vi "SetCalcSource.vi"(8 "error in (no error)":errorcluster caption="entrée d'erreur (pas d'erreur)", 9 "DataQRefs":refnum<queue>[](array[refnum]), 10 "ScanDataQ":string[](array[string]), 11 "InstrClassIn":refnum<class "Calculations.lvclass"> caption="DNL_LabVIEW Object in") -> (0 "error out":errorcluster caption="sortie d'erreur", 3 "InstrClassOut":refnum<class "Calculations.lvclass"> caption="DNL_LabVIEW Object out")   [LabVIEW 2019, in "Calculations.lvclass"]
uses:
  Calculations.lvclass
  Calculations.lvclass/Calculations.ctl
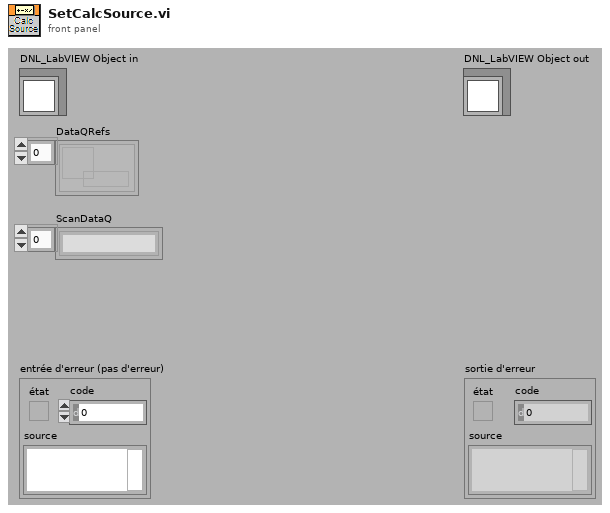
[diagram p1: front panel]
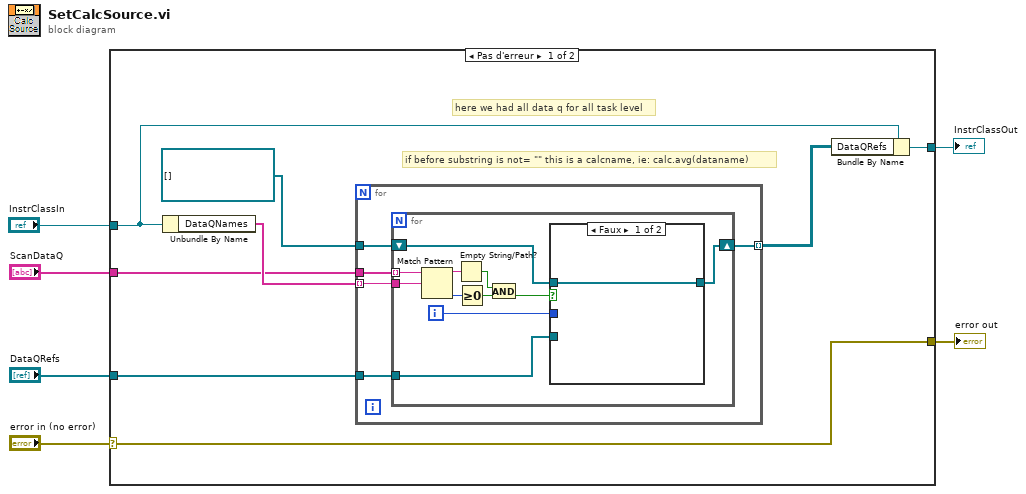
[diagram p0: block diagram]
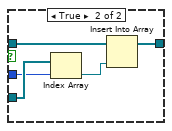
[diagram p2: hidden frame]
diagram:
  n1 = case shown="Pas d'erreur" "error in (no error)" {
    selector: "error in (no error)" -> [w7 w37]
    tunnel: "InstrClassIn" -> [w8 w38]
    tunnel: [w10 w38] -> w4
    tunnel: [w7 w37] -> w3
    tunnel: "ScanDataQ" -> [w13 _]
    tunnel: "DataQRefs" -> [w12 _]
    frame No Error {
      # "here we had all data q for all task level"
      # "if before substring is not= \"\" this is a calcname, ie: calc.avg(dataname)"
      n2 = Unbundle By Name(w8) -> ("DataQNames"=w14:string[])
      n3 = for {
        tunnel: w14 -> [w19] mode=indexing
        tunnel: w13 -> [w18]
        tunnel: w12 -> [w17]
        tunnel: refnum<queue>[] [] -> [w16]
        tunnel: [w15] -> w9 mode=indexing
        n4 = for {
          tunnel: w19 -> [w30]
          tunnel: w18 -> [w29] mode=indexing
          shift-right: [w24] -> w15
          shift-left: w16 -> [w23]
          tunnel: w17 -> [w26]
          i -> [w25]
          n5 = Match Pattern(string=w29, regular expression=w30) -> (before substring=w22:string, offset past match=w28:i32)  [unwired: 1 in, 2 out]
          n6 = Empty String/Path?(string/path=w22) -> (empty?=w20:bool)
          n7 = Greater Or Equal To 0?(x=w28) -> (x >= 0?=w27:bool)
          n8 = And(x=w20, y=w27) -> (x .and. y?=w21:bool)
          n9 = case shown="Faux" w21 {
            tunnel: w26 -> [_ w36]
            tunnel: w25 -> [_ w35]
            tunnel: [w31 w33] -> w24
            tunnel: w23 -> [w31 w32]
            frame False {
            }
            frame True {
              n10 = Index Array(array=w36, index=w35) -> (element=w34:refnum<queue>)
              n11 = Insert Into Array(array=w32, new element=w34) -> (w33:refnum<queue>[])  [unwired: 1 in]
            }
          }
        }
      }
      n12 = Bundle By Name(cluster=w8, "DataQRefs"=w9) -> (w10:refnum<class "Calculations.lvclass">)
    }
    frame Error {
    }
  }
  "error out" <- w3
  "InstrClassOut" <- w4
